vi "Read DC Pins.vi"(8 "error in (no error)":errorcluster, 11 "Harmonics in":refnum<class "Harmonics.lvclass">) -> (0 "error out":errorcluster, 2 "DC Pins":string[](array[string]), 3 "Harmonics out":refnum<class "Harmonics.lvclass">)   [LabVIEW 2016, in "Harmonics.lvlib" / "Harmonics.lvclass"]
uses:
  Harmonics.lvclass
  Harmonics.lvclass/Harmonics.ctl
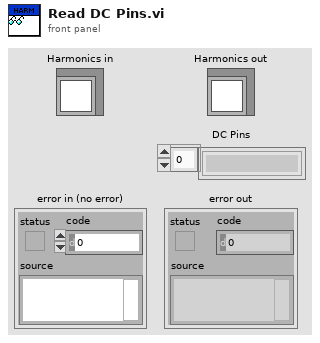
[diagram p1: front panel]
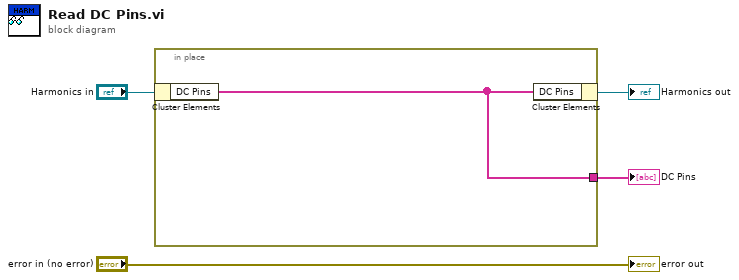
[diagram p0: block diagram]
diagram:
  n1 = in-place {
    in-place-border: [w5] -> w1
    n2 = in-place-cluster #1("Harmonics in") -> ("DC Pins"=w5:string[])
    n3 = in-place-cluster #1("DC Pins"=w5) -> (→"Harmonics out":refnum<class "Harmonics.lvclass">)
  }
  "DC Pins" <- w1
  "error out" <- "error in (no error)"
